vi "Fmix generate zmag.vi"(7 "exp fit":cluster{"A":dbl, "B":dbl}={"A"=28.47, "B"=-1.501}, 8 "阶段等待时间":dbl[](array[numeric]), 9 "阶段加载率":dbl[](array[numeric]), 10 "阶段终点":dbl[](array[numeric]), 11 "起点":dbl) -> (1 "FR time":dbl[](array[numeric]), 2 "FR zmag":dbl[](array[numeric]), 4 "Wrong":bool)   [LabVIEW 2017]
panel:
  in  "真 终点":dbl
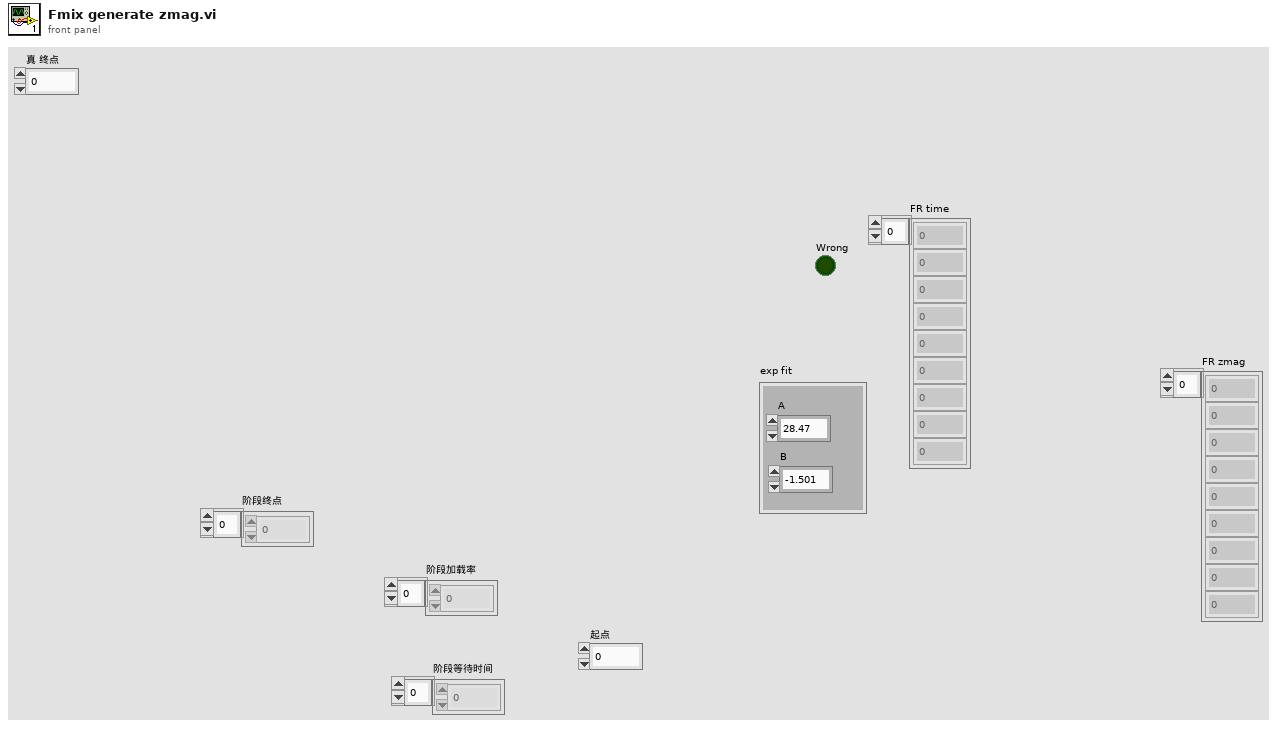
[diagram p1: front panel]
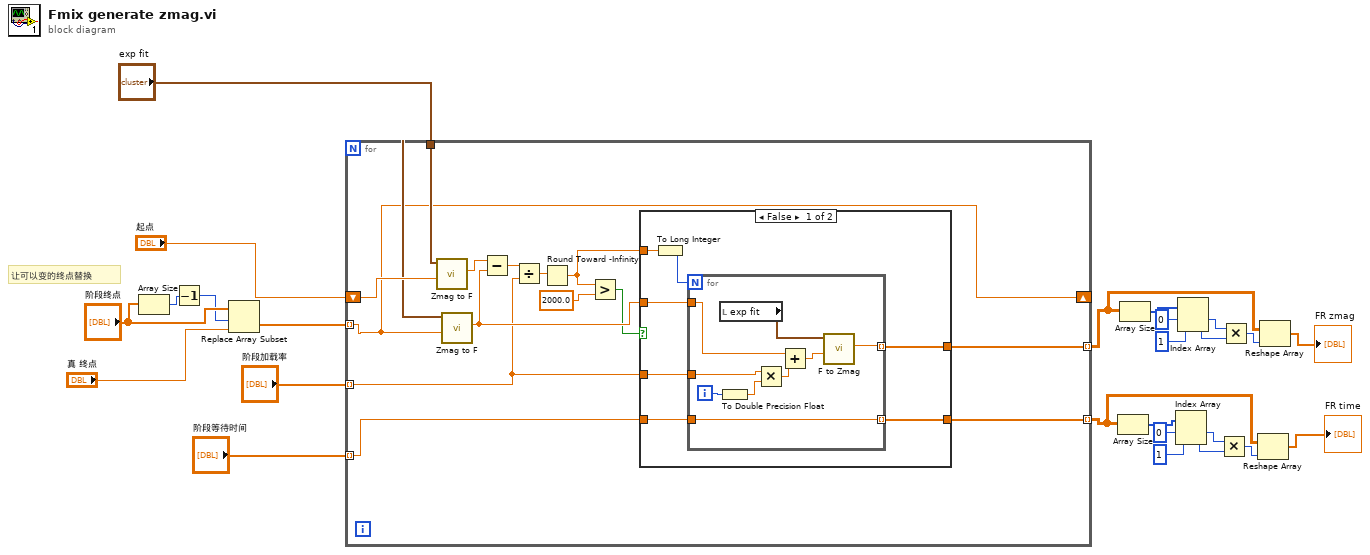
[diagram p0: block diagram]
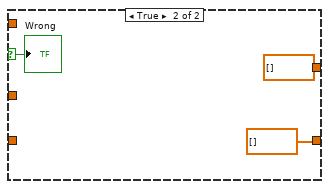
[diagram p2: hidden frame]
diagram:
  # "让可以变的终点替换"
  n1 = Array Size(array="阶段终点") -> (size(s)=w4:i32)
  n2 = Decrement(x=w4) -> (x-1=w2:i32)
  n3 = Replace Array Subset(array="阶段终点", new element="真 终点", index=w2) -> (w1:dbl[])
  n4 = for {
    tunnel: [w28] -> w16 mode=indexing
    tunnel: "exp fit" -> [w38]
    tunnel: "阶段加载率" -> [w27] mode=indexing
    tunnel: "阶段等待时间" -> [w30] mode=indexing
    tunnel: [w29] -> w7 mode=indexing
    shift-right: [w26] -> _
    shift-left: "起点" -> [w39]
    tunnel: w1 -> [w26] mode=indexing
    n5 = call "Zmag to F.vi"("Z 输入"=w39, "Parameter T1"=w38) -> ("F 输出"=w37:dbl)  [unwired: 9 in]
    n6 = call "Zmag to F.vi"("Z 输入"=w26, "Parameter T1"=w38) -> ("F 输出"=w36:dbl)  [unwired: 9 in]
    n7 = Subtract(x=w37, y=w36) -> (x-y=w35:dbl)
    n8 = Divide(x=w35, y=w27) -> (x/y=w34:dbl)
    n9 = Round Toward -Infinity(1:w34) -> (0:w33:dbl)
    n10 = Greater?(x=w33, y=2000.0) -> (0:w31:bool)
    n11 = case shown="False" w31 {
      selector: w31 -> [_ w57]
      tunnel: w36 -> [w46 _]
      tunnel: [w45 dbl[] []] -> w28
      tunnel: w33 -> [w44 _]
      tunnel: w30 -> [w43 _]
      tunnel: [w42 dbl[] []] -> w29
      tunnel: w27 -> [w40 _]
      frame False {
        n12 = To Long Integer(number=w44) -> (32bit integer=w41:i32)
        n13 = for {
          N: w41 -> [_]
          tunnel: w46 -> [w52]
          tunnel: [w50] -> w45 mode=indexing
          tunnel: w43 -> [w48]
          tunnel: [w48] -> w42 mode=indexing
          tunnel: w40 -> [w47]
          i -> [w55]
          n14 = local read "exp fit"() -> (w49:cluster{"A":dbl, "B":dbl})
          n15 = To Double Precision Float(number=w55) -> (double precision float=w54:dbl)
          n16 = Multiply(x=w47, y=w54) -> (x*y=w53:dbl)
          n17 = Add(x=w52, y=w53) -> (x+y=w51:dbl)
          n18 = call "F to Zmag.vi"("F输入"=w51, "Parameter T1"=w49) -> ("Z输出"=w50:dbl)  [unwired: 9 in]
        }
      }
      frame True {
        "Wrong" <- w57
      }
    }
  }
  n19 = Array Size(array=w7) -> (size(s)=w8:i32[])
  n20 = Array Size(array=w16) -> (size(s)=w21:i32[])
  n21 = Index Array(array=w8, index #1=0 ("index"), index #2=1 ("index")) -> (element #1=w11:i32, element #2=w12:i32)
  n22 = Index Array(array=w21, index #1=0 ("index"), index #2=1 ("index")) -> (element #1=w18:i32, element #2=w17:i32)
  n23 = Multiply(x=w11, y=w12) -> (x*y=w13:i32)
  n24 = Multiply(x=w18, y=w17) -> (x*y=w15:i32)
  n25 = Reshape Array(w7, w13) -> (→"FR time":dbl[])
  n26 = Reshape Array(w16, w15) -> (→"FR zmag":dbl[])
